vi "AWS-S3-ProcessUpload.vi"(0 "S3 Client ref":refnum<k24>, 5 "Put Object Request ref":refnum<k24>, 7 "Upload Complete":refnum<user-event>, 11 "error in":errorcluster) -> ()   [LabVIEW 2012, in "AWS-S3-API.lvclass"]
uses:
  AWS-S3-API.lvclass
  AWS-S3-Transfer-Header.ctl
  AWS-S3-Transfer-Completed.ctl
  C:/Users/Jack/repo/aws/AWS-SDK/AWSSDK.dll
  repo/aws/AWS-SDK/AWSSDK.dll
panel:
  # "Inputs"
  # "Outputs"
  # "No Outputs - this VI\nis fire and forget"
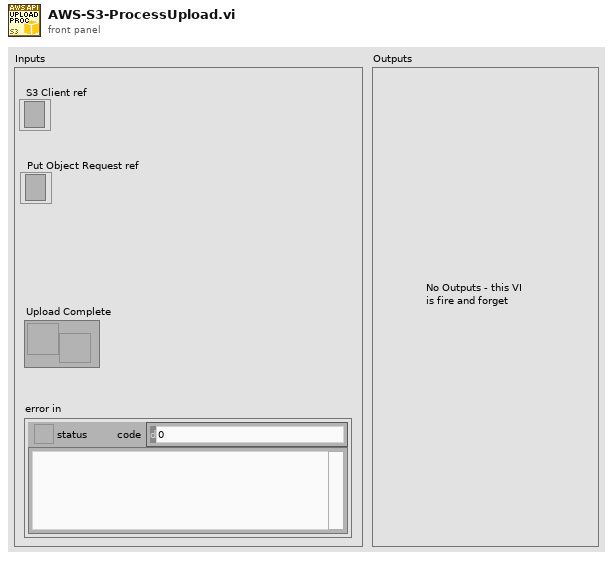
[diagram p1: front panel]
types:
  T1 = typedef "AWS-S3-API.lvclass/AWS-S3-Transfer-Completed.ctl" = cluster{"Transfer Header":T2, "Error?":bool, "Error Message":string}
  T2 = typedef "AWS-S3-API.lvclass/AWS-S3-Transfer-Header.ctl" = cluster{"Bucket Name":string, "Object Name":string, "Local Filepath":path}
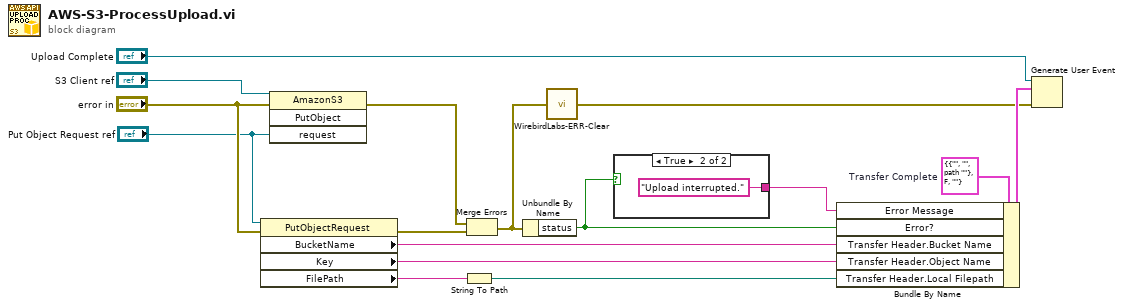
[diagram p0: block diagram]
diagram:
  w15 = T1 {"Transfer Header"={"Bucket Name"="", "Object Name"="", "Local Filepath"=path ""}, "Error?"=FALSE, "Error Message"=""}  # Transfer Complete
  n1 = property class="PutObjectRequest"(reference="Put Object Request ref", error in="error in") -> (error out=w7:errorcluster, "BucketName"=w13:string, "Key"=w12:string, "FilePath"=w11:string)  [unwired: 1 out]
  n2 = invoke class="AmazonS3" method="PutObject"(reference="S3 Client ref", error in="error in", "request"="Put Object Request ref") -> (error out=w8:errorcluster)  [unwired: 1 in, 3 out]
  n3 = String To Path(string=w11) -> (path=w10:path)
  n4 = Merge Errors(w8, w7) -> (w6:errorcluster)
  n5 = Unbundle By Name(w6) -> ("status"=w2:bool)
  n6 = call "WirebirdLabs-ERR-Clear.vi"("error to snuff"=w6) -> ("no error"=w5:errorcluster)
  n7 = case shown="True" w2 {
    tunnel: [_ "Upload interrupted." ("source")] -> w1
    frame False {
    }
    frame True {
    }
  }
  n8 = Bundle By Name(cluster=w15, "Error Message"=w1, "Error?"=w2, "Transfer Header.Bucket Name"=w13, "Transfer Header.Object Name"=w12, "Transfer Header.Local Filepath"=w10) -> (w14:T1)
  n9 = Generate User Event(user event="Upload Complete", event data cluster=w14, error in=w5) -> ()  [unwired: 2 out]
